vi "enumerateStaticDependencies.vi"(8 "error in (no error)":errorcluster, 11 "Instrument":refnum<class "Instrument.lvclass">) -> (0 "error out":errorcluster, 2 "Static Dependencies":refnum<class "Dependency.lvclass">[](array[class]), 3 "Instrument out":refnum<class "Instrument.lvclass">)   [LabVIEW 2016, in "Instrument.lvclass"]
doc: "JKI State Machine Objects (SMO) 1.3.0.56\nJKI - JKI\nCopyright (c) 2017, JKI"
uses:
  Instrument.lvclass
  <vilib>/JKI/JKI SMO/Dependency/Dependency.lvclass
  levylab_util_remote/src/RemoteControl/RemoteControl.lvclass
  C:/Program Files (x86)/National Instruments/LabVIEW 2016/vi.lib/JKI/JKI SMO/SMO/SMO.lvclass
  <vilib>/JKI/JKI SMO/SMO/SMO.lvclass
panel:
  # "For instructions on how to use the JKI State Machine Objects, examples and video tutorials, visit:\nhttp://jki.net/state-machine-objects/\n\nJKI State Machine Objects™\nhttp://jki.net/state-machine-objects/\nCopyright (C) 2005-2015, JKI <info@jki.net>\nALL RIGHTS RESERVED"
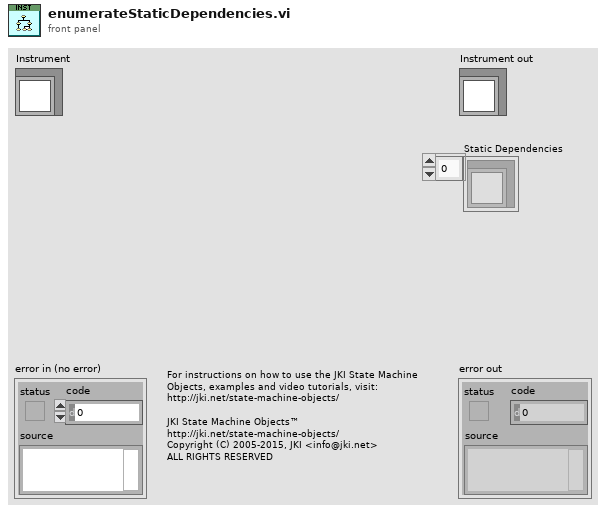
[diagram p1: front panel]
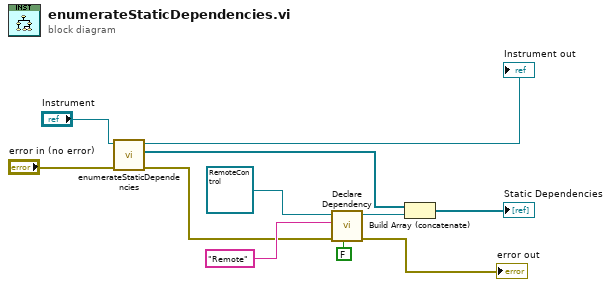
[diagram p0: block diagram]
diagram:
  n1 = call-parent "enumerateStaticDependencies.vi"("error in (no error)"="error in (no error)", "SMO"="Instrument") -> ("error out"=w2:errorcluster, "Static Dependencies"=w6:refnum<class "Dependency.lvclass">[], "SMO out"=→"Instrument out":refnum<class "Instrument.lvclass">)  [unwired: 7 in]
  n2 = call <vilib>:"Declare Dependency.vi"("Shared Resource (F)"=FALSE, "error in (no error)"=w2, "Name"="Remote", "Type"=refnum<class "RemoteControl.lvclass"> refnum ("RemoteControl.lvclass")) -> ("error out"=→"error out":errorcluster, "Dependency out"=w7:refnum<class "Dependency.lvclass">)  [unwired: 6 in]
  n3 = Build Array (concatenate)(w6, w7) -> (→"Static Dependencies":refnum<class "Dependency.lvclass">[])
